vi "Save Load String.vi"(7 "Name":string, 8 "error in":errorcluster, 10 "String (in)":string, 11 "Save Load Info (in)":T1) -> (0 "error out":errorcluster, 2 "String (out)":string, 3 "Save Load Info (out)":T1)   [LabVIEW 2016]
uses:
  Load Save Info.ctl
  <vilib>/Utility/config.llb/Config Data RefNum.ctl
  <vilib>/Rock Robotics/Network Tables/NT Write String.vi
  <vilib>/Utility/config.llb/Write Key (String).vi
  <vilib>/Rock Robotics/Network Tables/NT Read String.vi
  <vilib>/Utility/config.llb/Read Key (String).vi
  <vilib>/Utility/config.llb/NI_LVConfig.lvlib
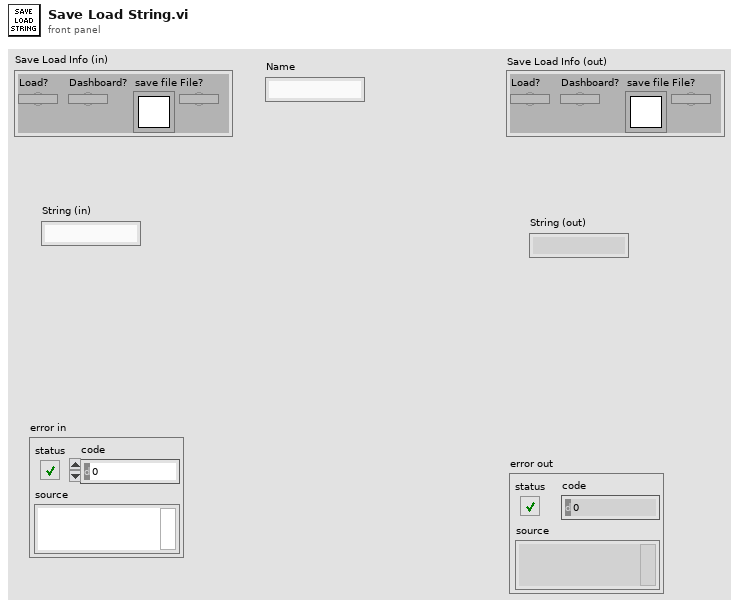
[diagram p1: front panel]
types:
  T1 = typedef "Load Save Info.ctl" = cluster{"Load?":bool, "Dashboard?":bool, "save file":T2, "File?":bool}
  T2 = typedef "NI_LVConfig.lvlib/Config Data RefNum.ctl" = refnum<k1>
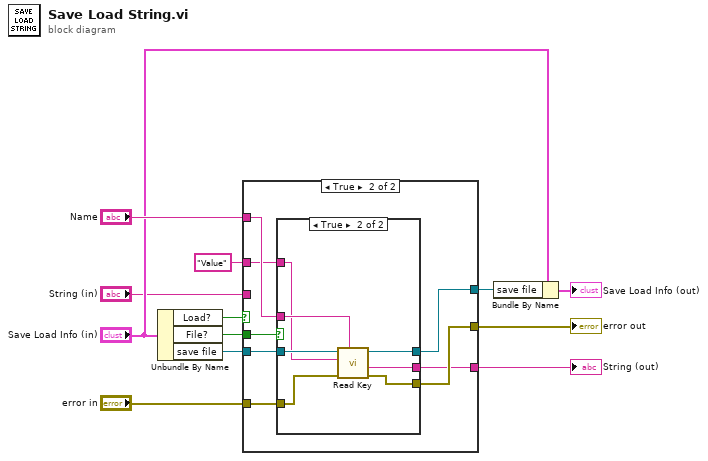
[diagram p0: block diagram]
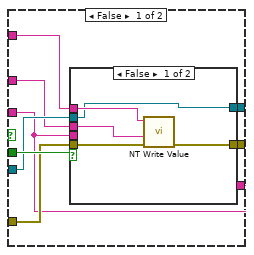
[diagram p2: hidden frame]
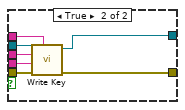
[diagram p3: hidden frame]
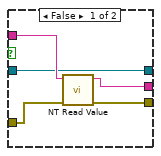
[diagram p4: hidden frame]
diagram:
  n1 = Unbundle By Name("Save Load Info (in)") -> ("Load?"=w12:bool, "File?"=w11:bool, "save file"=w8:T2)
  n2 = case shown="True" w12 {
    tunnel: w11 -> [w20 w40]
    tunnel: "Name" -> [w19 w37]
    tunnel: "String (in)" -> [w13 _]
    tunnel: "error in" -> [w18 w39]
    tunnel: w8 -> [w17 w38]
    tunnel: [w16 w35] -> w7
    tunnel: [w15 w36] -> w4
    tunnel: [w13 w34] -> w1
    tunnel: "Value" ("key") -> [w14 w33]
    frame False {
      n3 = case shown="False" w20 {
        tunnel: w19 -> [w25 w31]
        tunnel: w18 -> [w24 w32]
        tunnel: [w23 w30] -> w15
        tunnel: w17 -> [w22 w29]
        tunnel: [w22 w28] -> w16
        tunnel: w14 -> [w21 w27]
        tunnel: w13 -> [_ w26]
        frame False {
          n4 = call-poly <vilib>:"NT Write Value.vi"("error in"=w24, "String"=w21, "Name"=w25) -> ("error out"=w23:errorcluster)  [unwired: 8 in]
        }
        frame True {
          n5 = call-poly <vilib>:"Write Key.vi"("section"=w31, "error in (no error)"=w32, "value"=w26, "key"=w27, "refnum"=w29) -> ("error out"=w30:errorcluster, "refnum out"=w28:T2)  [unwired: 4 in, 1 out]
        }
      }
    }
    frame True {
      n6 = case shown="True" w40 {
        tunnel: w39 -> [w45 w52]
        tunnel: w38 -> [w42 w51]
        tunnel: w37 -> [w43 w50]
        tunnel: [w44 w49] -> w36
        tunnel: [w42 w48] -> w35
        tunnel: [w41 w47] -> w34
        tunnel: w33 -> [_ w46]
        frame False {
          n7 = call-poly <vilib>:"NT Read Value.vi"("error in"=w45, "Name"=w43) -> ("error out"=w44:errorcluster, "String"=w41:string)  [unwired: 8 in]
        }
        frame True {
          n8 = call-poly <vilib>:"Read Key.vi"("section"=w50, "error in (no error)"=w52, "key"=w46, "refnum"=w51) -> ("error out"=w49:errorcluster, "value"=w47:string, "refnum out"=w48:T2)  [unwired: 4 in, 1 out]
        }
      }
    }
  }
  "error out" <- w4
  "String (out)" <- w1
  n9 = Bundle By Name(cluster="Save Load Info (in)", "save file"=w7) -> (→"Save Load Info (out)":T1)
